vi "BMU参数读取-Auto.vi"(7 "Socket":dbl, 8 "CAN端口":u16(ring), 9 "设备索引号":u16(ring), 10 "CAN卡类型":u32(ring)=21, 11 "从板号":u8=1) -> (3 "成功?":bool)   [LabVIEW 2013] (continued)
                n1579 = Wait Until Next ms Multiple(millisecond multiple=u32 100 ("毫秒倍数")) -> ()  [unwired: 1 out]
              }
            }
            frame #2 {
              n1580 = case shown="真" w2578 {
                frame False {
                  n1581 = Concatenate Strings("故障信息" ("字符串"), "     读取失败" ("字符串")) -> (w2580:string)
                  n1582 = One Button Dialog(message=w2580, button name ("OK")="确定" ("按钮名称（“确定”）")) -> ()  [unwired: 1 out]
                }
                frame True {
                  n1583 = One Button Dialog(message="故障信息读取完成" ("字符串"), button name ("OK")="确定" ("按钮名称（“确定”）")) -> ()  [unwired: 1 out]
                }
              }
              n1584 = call <vilib>:"Unset Busy.vi"() -> ()  [unwired: 2 in, 10 out]
            }
          }
        }
        frame "平台软件版本读取" {
          n1585 = stacked-sequence {
            seq-local: [_ w2600 _] -> [_ _ w2607]
            frame #0 {
              n1586 = local read "设备索引号"() -> (w2587:u16)
              n1587 = local read "CAN卡类型"() -> (w2588:u32)
              n1588 = local read "CAN端口"() -> (w2586:u16)
              n1589 = stacked-sequence {
                tunnel: w2588 -> [w2591 w2599]
                tunnel: w2587 -> [w2590 w2598]
                tunnel: w2586 -> [w2589 w2597]
                tunnel: u8 137 ("命令") -> [_ w2596]
                frame #0 {
                  n1590 = dll-call lib="PTH1abs FBluewave New EnergySVN_WorkAutoTest_TestStandtrunkAutoTest_TestStandDriverZlgCanBHN01è¯»ååæ°data\nkerneldlls\nusbcan.dll" fn="VCI_ClearBuffer"("DeviceType"=w2591, "DeviceInd"=w2590, "CANInd"=w2589) -> (error out=w2592:errorcluster)  [unwired: 4 in, 4 out]
                  n1591 = call <vilib>:"Clear Errors.vi"("error in (no error)"=w2592) -> ()  [unwired: 6 in, 1 out]
                }
                frame #1 {
                  w2595 = u32 2 ("命令序号")
                  n1592 = local read "从板板号"() -> (w2593:u8)
                  n1593 = local write "命令"(w2596) -> ()
                  n1594 = call "多帧发送机制(EV05).vi"("can卡类型"=w2599, "设备索引号"=w2598, "CAN端口"=w2597, "命令"=w2596, "板号"=w2593, "命令序号"=w2595, "输入数据"=dbl[] [0.0]) -> ()  [unwired: 2 in, 11 out]
                  n1595 = local write "命令序号"(w2595) -> ()
                }
              }
            }
            frame #1 {
              n1596 = while {
                tunnel: [w2601] -> w2600
                i -> [w2606]
                stop <- w2603 stop-if-true
                n1597 = global read "EV05全局变量1.vi" "写入超时"() -> (w2601:bool)
                n1598 = Greater Or Equal?(x=w2606, y=25) -> (x >= y?=w2604:bool)
                n1599 = Or(x=w2601, y=w2604) -> (x .or. y?=w2603:bool)
                n1600 = Wait Until Next ms Multiple(millisecond multiple=u32 100 ("毫秒倍数")) -> ()  [unwired: 1 out]
              }
            }
            frame #2 {
              n1601 = case shown="假" w2607 {
                frame False {
                  n1602 = control-ref of="结果"() -> (w2610:refnum<vi>)
                  n1603 = Concatenate Strings("平台软件版本" ("字符串"), "     读取失败" ("字符串")) -> (w2612:string)
                  n1604 = Build Array(w2612) -> (w2609:string[])
                  n1605 = call "表格编辑(版本读取).vi"("新元素/子数组"=w2609, "活动单元格:单元格背景色"=u32 16740749, "MCListbox引用句柄"=w2610) -> ()  [unwired: 9 out]
                }
                frame True {
                }
              }
              n1606 = call <vilib>:"Unset Busy.vi"() -> ()  [unwired: 2 in, 10 out]
            }
          }
        }
        frame "模块软件版本读取" {
          n1607 = local read "从板板号"() -> (w2614:u8)
          n1608 = local read "模块软件版本"() -> (w2615:T1)
          n1609 = case shown="\"全部读取\"" w2615 {
            selector: w2615 -> [w2616 w2660]
            tunnel: w2614 -> [_ w2659]
            frame "BCUMCAL", Default {
              n1610 = stacked-sequence {
                seq-local: [_ _ w2642 _] -> [_ _ _ w2649]
                tunnel: w2616 -> [_ w2622 _ w2650]
                frame #0 {
                  w2621 = FALSE ("写?")
                  n1611 = call <vilib>:"Set Busy.vi"("disable click? (T)"=FALSE) -> ()  [unwired: 3 in, 8 out]
                  n1612 = local write "写?"(w2621) -> ()
                  n1613 = global write "EV05全局变量1.vi" "流控帧 2"(TRUE ("流控帧 2")) -> ()
                  n1614 = global write "EV05全局变量1.vi" "写入超时"(w2621) -> ()
                  n1615 = local write "控制1"(TRUE ("控制1")) -> ()
                  n1616 = local write "消除"(TRUE ("消除")) -> ()
                }
                frame #1 {
                  n1617 = Quotient & Remainder(x=w2622, y=256) -> (x-y*floor(x/y)=w2623:i32, floor(x/y)=w2624:i32)
                  n1618 = Build Array(w2624, w2623, u8 0 ("板号")) -> (w2627:i32[])
                  n1619 = local read "设备索引号"() -> (w2629:u16)
                  n1620 = local read "CAN卡类型"() -> (w2630:u32)
                  n1621 = local read "CAN端口"() -> (w2628:u16)
                  n1622 = stacked-sequence {
                    tunnel: w2630 -> [w2633 w2641]
                    tunnel: w2629 -> [w2632 w2640]
                    tunnel: w2628 -> [w2631 w2639]
                    tunnel: w2627 -> [_ w2638]
                    frame #0 {
                      n1623 = dll-call lib="PTH1abs FBluewave New EnergySVN_WorkAutoTest_TestStandtrunkAutoTest_TestStandDriverZlgCanBHN01è¯»ååæ°data\nkerneldlls\nusbcan.dll" fn="VCI_ClearBuffer"("DeviceType"=w2633, "DeviceInd"=w2632, "CANInd"=w2631) -> (error out=w2634:errorcluster)  [unwired: 4 in, 4 out]
                      n1624 = call <vilib>:"Clear Errors.vi"("error in (no error)"=w2634) -> ()  [unwired: 6 in, 1 out]
                    }
                    frame #1 {
                      w2637 = u8 137 ("命令")
                      w2635 = u32 3 ("命令序号")
                      n1625 = local read "从板板号"() -> (w2636:u8)
                      n1626 = local write "命令"(w2637) -> ()
                      n1627 = call "多帧发送机制(EV05).vi"("can卡类型"=w2641, "设备索引号"=w2640, "CAN端口"=w2639, "命令"=w2637, "板号"=w2636, "命令序号"=w2635, "输入数据"=w2638) -> ()  [unwired: 2 in, 11 out]
                      n1628 = local write "命令序号"(w2635) -> ()
                    }
                  }
                }
                frame #2 {
                  n1629 = while {
                    tunnel: [w2643] -> w2642
                    i -> [w2648]
                    stop <- w2644 stop-if-true
                    n1630 = global read "EV05全局变量1.vi" "写入超时"() -> (w2643:bool)
                    n1631 = Greater Or Equal?(x=w2648, y=25) -> (x >= y?=w2645:bool)
                    n1632 = Or(x=w2643, y=w2645) -> (x .or. y?=w2644:bool)
                    n1633 = Wait Until Next ms Multiple(millisecond multiple=u32 100 ("毫秒倍数")) -> ()  [unwired: 1 out]
                  }
                }
                frame #3 {
                  n1634 = call <vilib>:"Unset Busy.vi"() -> ()  [unwired: 2 in, 10 out]
                  n1635 = case shown="假" w2649 {
                    tunnel: w2650 -> [w2652 _]
                    frame False {
                      n1636 = Number To Decimal String(number=w2652) -> (decimal integer string=w2653:string)  [unwired: 1 out]
                      n1637 = control-ref of="结果"() -> (w2654:refnum<vi>)
                      n1638 = Concatenate Strings("模块" ("字符串"), w2653, "     读取失败" ("字符串")) -> (w2657:string)
                      n1639 = Build Array(w2657) -> (w2656:string[])
                      n1640 = call "表格编辑(版本读取).vi"("新元素/子数组"=w2656, "活动单元格:单元格背景色"=u32 16740749, "MCListbox引用句柄"=w2654) -> ()  [unwired: 9 out]
                    }
                    frame True {
                    }
                  }
                }
              }
            }
            frame "全部读取" {
              n1641 = stacked-sequence {
                seq-local: [w2661 _] -> [_ w2699]
                tunnel: w2660 -> [_ w2701]
                tunnel: w2659 -> [w2662 w2700]
                frame #0 {
                  n1642 = stacked-sequence {
                    tunnel: w2662 -> [_ w2671 _]
                    tunnel: [_ _ w2691] -> w2661
                    frame #0 {
                      w2667 = FALSE ("写?")
                      n1643 = control-ref of="模块软件版本 2"() -> (w2665:refnum<vi>)
                      n1644 = call <vilib>:"Set Busy.vi"("disable click? (T)"=FALSE) -> ()  [unwired: 3 in, 8 out]
                      n1645 = local write "写?"(w2667) -> ()
                      n1646 = property class="MCListbox (严格)"(reference=w2665, "ItemNames"=string[][] []) -> ()  [unwired: 1 in, 2 out]
                      n1647 = global write "EV05全局变量1.vi" "写入超时"(w2667) -> ()
                      n1648 = local write "消除"(TRUE ("消除")) -> ()
                      n1649 = global write "EV05全局变量1.vi" "流控帧 2"(TRUE ("流控帧 2")) -> ()
                      n1650 = local write "控制1"(TRUE ("控制1")) -> ()
                      n1651 = local write "MODEL号"(u8[] [] ("MODEL号")) -> ()
                    }
                    frame #1 {
                      n1652 = local read "设备索引号"() -> (w2673:u16)
                      n1653 = local read "CAN卡类型"() -> (w2674:u32)
                      n1654 = local read "CAN端口"() -> (w2672:u16)
                      n1655 = stacked-sequence {
                        tunnel: w2674 -> [w2677 w2690]
                        tunnel: w2673 -> [w2676 w2689]
                        tunnel: w2672 -> [w2675 w2688]
                        tunnel: w2671 -> [_ w2680]
                        frame #0 {
                          n1656 = dll-call lib="PTH1abs FBluewave New EnergySVN_WorkAutoTest_TestStandtrunkAutoTest_TestStandDriverZlgCanBHN01è¯»ååæ°data\nkerneldlls\nusbcan.dll" fn="VCI_ClearBuffer"("DeviceType"=w2677, "DeviceInd"=w2676, "CANInd"=w2675) -> (error out=w2678:errorcluster)  [unwired: 4 in, 4 out]
                          n1657 = call <vilib>:"Clear Errors.vi"("error in (no error)"=w2678) -> ()  [unwired: 6 in, 1 out]
                        }
                        frame #1 {
                          w2686 = u8 137 ("命令")
                          w2684 = u32 3 ("命令序号")
                          n1658 = Quotient & Remainder(x=u8 0 ("板号"), y=256) -> (x-y*floor(x/y)=w2681:i32, floor(x/y)=w2682:i32)
                          n1659 = local write "命令"(w2686) -> ()
                          n1660 = Build Array(w2682, w2681, u8 0 ("板号")) -> (w2687:i32[])
                          n1661 = call "多帧发送机制(EV05).vi"("can卡类型"=w2690, "设备索引号"=w2689, "CAN端口"=w2688, "命令"=w2686, "板号"=w2680, "命令序号"=w2684, "输入数据"=w2687) -> ()  [unwired: 2 in, 11 out]
                          n1662 = local write "命令序号"(w2684) -> ()
                        }
                      }
                    }
                    frame #2 {
                      n1663 = while {
                        tunnel: [w2693] -> w2691
                        i -> [w2697]
                        stop <- w2694 stop-if-true
                        n1664 = local read "强制停止版本读取"() -> (w2692:bool)
                        n1665 = global read "EV05全局变量1.vi" "写入超时"() -> (w2693:bool)
                        n1666 = Greater Or Equal?(x=w2697, y=35) -> (x >= y?=w2695:bool)
                        n1667 = Compound Arithmetic op=OR(w2692, w2693, w2695) -> (w2694:bool)
                        n1668 = Wait Until Next ms Multiple(millisecond multiple=u32 100 ("毫秒倍数")) -> ()  [unwired: 1 out]
                      }
                    }
                  }
                }
                frame #1 {
                  n1669 = case shown="真" w2699 {
                    tunnel: w2701 -> [_ w2711]
                    tunnel: w2700 -> [_ w2710]
                    frame False {
                      n1670 = control-ref of="结果"() -> (w2703:refnum<vi>)
                      n1671 = Concatenate Strings("模块编号" ("字符串"), "读取失败" ("字符串")) -> (w2706:string)
                      n1672 = Build Array(w2706) -> (w2705:string[])
                      n1673 = call "表格编辑(版本读取).vi"("新元素/子数组"=w2705, "活动单元格:单元格背景色"=u32 16740749, "MCListbox引用句柄"=w2703) -> ()  [unwired: 9 out]
                      n1674 = call <vilib>:"Unset Busy.vi"() -> ()  [unwired: 11 in, 1 out]
                    }
                    frame True {
                      n1675 = local read "MODEL号"() -> (w2709:u8[])
                      n1676 = Array Size(array=w2709) -> (size(s)=w2708:i32)
                      n1677 = for {
                        tunnel: w2711 -> [_]
                        tunnel: w2710 -> [w2714]
                        tunnel: w2709 -> [w2713] mode=indexing
                        tunnel: w2708 -> [w2712]
                        i -> [w2716]
                        n1678 = Increment(x=w2716) -> (x+1=w2715:i32)
                        n1679 = stacked-sequence {
                          seq-local: [_ _ _ w2743 _ _] -> [_ _ _ _ w2752 _]
                          seq-local: [_ w2722 _ _ _ _] -> [_ _ _ _ w2751 _]
                          tunnel: w2715 -> [_ _ _ _ _ w2763]
                          tunnel: w2713 -> [_ w2722 _ _ _ _]
                          tunnel: w2714 -> [_ w2723 _ _ _ _]
                          tunnel: w2712 -> [_ _ _ _ _ w2761]
                          frame #0 {
                            w2718 = FALSE ("写?")
                            n1680 = call <vilib>:"Set Busy.vi"("disable click? (T)"=FALSE) -> ()  [unwired: 3 in, 8 out]
                            n1681 = local write "写?"(w2718) -> ()
                            n1682 = global write "EV05全局变量1.vi" "写入超时"(w2718) -> ()
                            n1683 = global write "EV05全局变量1.vi" "流控帧 2"(TRUE ("流控帧 2")) -> ()
                            n1684 = local write "控制1"(TRUE ("控制1")) -> ()
                            n1685 = local write "消除"(TRUE ("消除")) -> ()
                          }
                          frame #1 {
                            n1686 = local read "设备索引号"() -> (w2725:u16)
                            n1687 = local read "CAN卡类型"() -> (w2726:u32)
                            n1688 = local read "CAN端口"() -> (w2724:u16)
                            n1689 = stacked-sequence {
                              tunnel: w2726 -> [w2729 w2742]
                              tunnel: w2725 -> [w2728 w2741]
                              tunnel: w2724 -> [w2727 w2740]
                              tunnel: w2723 -> [_ w2732]
                              tunnel: w2722 -> [_ w2731]
                              frame #0 {
                                n1690 = dll-call lib="PTH1abs FBluewave New EnergySVN_WorkAutoTest_TestStandtrunkAutoTest_TestStandDriverZlgCanBHN01è¯»ååæ°data\nkerneldlls\nusbcan.dll" fn="VCI_ClearBuffer"("DeviceType"=w2729, "DeviceInd"=w2728, "CANInd"=w2727) -> (error out=w2730:errorcluster)  [unwired: 4 in, 4 out]
                                n1691 = call <vilib>:"Clear Errors.vi"("error in (no error)"=w2730) -> ()  [unwired: 6 in, 1 out]
                              }
                              frame #1 {
                                w2738 = u8 137 ("命令")
                                w2736 = u32 3 ("命令序号")
                                n1692 = Quotient & Remainder(x=w2731, y=256) -> (x-y*floor(x/y)=w2733:i32, floor(x/y)=w2734:i32)
                                n1693 = local write "命令"(w2738) -> ()
                                n1694 = Build Array(w2734, w2733, u8 0 ("板号")) -> (w2739:i32[])
                                n1695 = call "多帧发送机制(EV05).vi"("can卡类型"=w2742, "设备索引号"=w2741, "CAN端口"=w2740, "命令"=w2738, "板号"=w2732, "命令序号"=w2736, "输入数据"=w2739) -> ()  [unwired: 2 in, 11 out]
                                n1696 = local write "命令序号"(w2736) -> ()
                              }
                            }
                          }
                          frame #2 {
                          }
                          frame #3 {
                            n1697 = while {
                              tunnel: [w2745] -> w2743
                              i -> [w2749]
                              stop <- w2746 stop-if-true
                              n1698 = local read "强制停止版本读取"() -> (w2744:bool)
                              n1699 = global read "EV05全局变量1.vi" "写入超时"() -> (w2745:bool)
                              n1700 = Greater Or Equal?(x=w2749, y=25) -> (x >= y?=w2747:bool)
                              n1701 = Compound Arithmetic op=OR(w2744, w2745, w2747) -> (w2746:bool)
                              n1702 = Wait Until Next ms Multiple(millisecond multiple=u32 100 ("毫秒倍数")) -> ()  [unwired: 1 out]
                            }
                          }
                          frame #4 {
                            n1703 = call <vilib>:"Unset Busy.vi"() -> ()  [unwired: 11 in, 1 out]
                            n1704 = case shown="假" w2752 {
                              tunnel: w2751 -> [w2754 _]
                              frame False {
                                n1705 = control-ref of="结果"() -> (w2756:refnum<vi>)
                                n1706 = Number To Decimal String(number=w2754) -> (decimal integer string=w2755:string)  [unwired: 1 out]
                                n1707 = Concatenate Strings("模块" ("字符串"), w2755, "     读取失败" ("字符串")) -> (w2759:string)
                                n1708 = Build Array(w2759) -> (w2758:string[])
                                n1709 = call "表格编辑(版本读取).vi"("新元素/子数组"=w2758, "活动单元格:单元格背景色"=u32 16740749, "MCListbox引用句柄"=w2756) -> ()  [unwired: 9 out]
                              }
                              frame True {
                              }
                            }
                          }
                          frame #5 {
                            n1710 = Equal?(x=w2761, y=w2763) -> (x = y?=w2762:bool)
                            n1711 = case shown="真" w2762 {
                              frame False {
                              }
                              frame True {
                                n1712 = control-ref of="模块软件版本 2"() -> (w2774:refnum<vi>)
                                n1713 = local read "模块版本名称"() -> (w2773:string[][])
                                n1714 = local read "模块版本值"() -> (w2769:string[][])
                                n1715 = control-ref of="结果"() -> (w2781:refnum<vi>)
                                n1716 = property class="MCListbox (严格)"(reference=w2774) -> ("ItemNames"=w2777:string[][])  [unwired: 1 in, 2 out]
                                n1717 = local read "从板板号"() -> (w2764:u8)
                                n1718 = Concatenate Strings("模块版本读取完成" ("字符串")) -> (w2784:string)
                                n1719 = Build Array(w2784) -> (w2783:string[])
                                n1720 = call "表格编辑(版本读取).vi"("新元素/子数组"=w2783, "活动单元格:单元格背景色"=u32 21937, "MCListbox引用句柄"=w2781) -> ()  [unwired: 9 out]
                                n1721 = Transpose 2D Array(2D array=w2777) -> (transposed array=w2778:string[][])
                                n1722 = local write "强制停止版本读取"(FALSE ("强制停止 2")) -> ()
                                n1723 = local read "模块个数"() -> (w2767:u8[])
                                n1724 = Index Array(array=w2778, index (row) #1=0 ("索引 (行)"), index (row) #2=1 ("索引 (行)")) -> (element #1=w2768:string[], element #2=w2770:string[])  [unwired: 2 in]
                                n1725 = Replace Array Subset(array=w2773, new element=w2768, index (row)=w2764) -> (w2772:string[][])  [unwired: 1 in]
                                n1726 = Replace Array Subset(array=w2769, new element=w2770, index (row)=w2764) -> (w2771:string[][])  [unwired: 1 in]
                                n1727 = local write "模块版本名称"(w2772) -> ()
                                n1728 = local write "模块版本值"(w2771) -> ()
                                n1729 = Array Size(array=w2768) -> (size(s)=w2765:i32)
                                n1730 = Replace Array Subset(array=w2767, new element=w2765, index=w2764) -> (w2766:u8[])
                                n1731 = local write "模块个数"(w2766) -> ()
                              }
                            }
                          }
                        }
                      }
                    }
                  }
                }
              }
            }
          }
        }
        frame "硬件版本读取" {
          n1732 = stacked-sequence {
            seq-local: [_ _ w2792 _] -> [_ _ _ w2799]
            frame #0 {
              w2788 = u8 137 ("命令")
              w2787 = u32 4 ("命令序号")
              n1733 = local read "设备索引号"() -> (w2790:u16)
              n1734 = local read "CAN卡类型"() -> (w2791:u32)
              n1735 = local read "CAN端口"() -> (w2789:u16)
              n1736 = local read "从板板号"() -> (w2785:u8)
              n1737 = local write "命令"(w2788) -> ()
              n1738 = call "多帧发送机制(EV05).vi"("can卡类型"=w2791, "设备索引号"=w2790, "CAN端口"=w2789, "命令"=w2788, "板号"=w2785, "命令序号"=w2787, "输入数据"=dbl[] [0.0]) -> ()  [unwired: 2 in, 11 out]
              n1739 = local write "命令序号"(w2787) -> ()
            }
            frame #1 {
            }
            frame #2 {
              n1740 = while {
                tunnel: [w2793] -> w2792
                i -> [w2798]
                stop <- w2794 stop-if-true
                n1741 = global read "EV05全局变量1.vi" "写入超时"() -> (w2793:bool)
                n1742 = Greater Or Equal?(x=w2798, y=25) -> (x >= y?=w2795:bool)
                n1743 = Or(x=w2793, y=w2795) -> (x .or. y?=w2794:bool)
                n1744 = Wait Until Next ms Multiple(millisecond multiple=u32 100 ("毫秒倍数")) -> ()  [unwired: 1 out]
              }
            }
            frame #3 {
              n1745 = case shown="假" w2799 {
                frame False {
                  n1746 = control-ref of="结果"() -> (w2801:refnum<vi>)
                  n1747 = Concatenate Strings("硬件版本" ("字符串"), "     读取失败" ("字符串")) -> (w2804:string)
                  n1748 = Build Array(w2804) -> (w2803:string[])
                  n1749 = call "表格编辑(版本读取).vi"("新元素/子数组"=w2803, "活动单元格:单元格背景色"=u32 16740749, "MCListbox引用句柄"=w2801) -> ()  [unwired: 9 out]
                }
                frame True {
                }
              }
              n1750 = call <vilib>:"Unset Busy.vi"() -> ()  [unwired: 2 in, 10 out]
            }
          }
        }
        frame "写配置文件" {
          n1751 = disable-structure shown="启用" {
            frame Enabled {
              n1752 = local read "主从选择"() -> (w2813:enum32{"主板", "从板"})
              n1753 = case shown="\"主板\", 默认" w2813 {
                tunnel: [w2832 w3023] -> w2816
                tunnel: ["M0" w3029] -> w2814
                frame "主板", Default {
                  n1754 = stacked-sequence {
                    seq-local: [w2846 _ _ _ _ _ _] -> [_ w2876 _ _ _ _ _]
                    seq-local: [string[] ["电池额定容量", "电池实际容量", "SOC", "SOH", "车牌号", "配置文件版本", "产品编号", "系统时钟"] _ _ _ _ _ _] -> [_ w2871 _ _ _ _ _]
                    seq-local: [_ _ _ _ string[] ["风机开启温度", "风机关闭温度", "加热开启温度", "加热关闭温度", "风机开启温差", "风机关闭温差", "加热关闭温差"] _ _] -> [_ _ _ _ _ w2975 _]
                    seq-local: [_ _ _ _ w2956 _ _] -> [_ _ _ _ _ w2973 _]
                    tunnel: [w2847 _ _ _ _ _ _] -> w2834
                    tunnel: [_ w2870 _ _ _ _ _] -> w2831
                    tunnel: [_ _ w2901 _ _ _ _] -> w2830
                    tunnel: [_ _ _ w2928 _ _ _] -> w2829
                    tunnel: [_ _ _ _ _ w2976 _] -> w2828
                    tunnel: [_ _ _ _ _ _ w2993] -> w2827
                    frame #0 {
                      w2838 = string[] ["", "", "", "", "", "", "", "", "", "", "  ", "", "", "", "", "", "", "", "", "", "  "]
                      n1755 = control-ref of="项目信息"() -> (w2866:refnum<vi>)
                      n1756 = property class="Tbl (严格)"(reference=w2866) -> ("Value"=w2842:string[][])  [unwired: 1 in, 2 out]
                      n1757 = control-ref of="项目信息2"() -> (w2860:refnum<vi>)
                      n1758 = Index Array(array=w2842, index (col)=0 ("禁用的索引 (列)")) -> (element=w2843:string[])  [unwired: 1 in]
                      n1759 = property class="Clust (严格)"(reference=w2860) -> ("Value"=w2859:T10)  [unwired: 1 in, 2 out]
                      n1760 = Index Array(array=w2842, index (col)=1 ("禁用的索引 (列)")) -> (element=w2841:string[])  [unwired: 1 in]
                      n1761 = local read "从板个数"() -> (w2865:dbl)
                      n1762 = Number To Decimal String(number=w2865) -> (decimal integer string=w2864:string)  [unwired: 1 out]
                      n1763 = Insert Into Array(array=w2843, new element=w2838) -> (w2840:string[])  [unwired: 1 in]
                      n1764 = Insert Into Array(array=w2841, new element=w2838) -> (w2839:string[])  [unwired: 1 in]
                      n1765 = Unbundle(w2859) -> ("电池额定容量(A)"=w2858:dbl, "电池实际容量(A)"=w2857:dbl, "车架(牌)号"=w2855:string, "配置文件版本"=w2854:string, "SOH(%)"=w2849:dbl, "SOC(%)"=w2848:dbl, "产品编号"=w2853:string, "系统时钟"=w2852:string)  [unwired: 1 out]
                      n1766 = Build Array("从板个数" ("元素"), w2864) -> (w2861:string[])
                      n1767 = Build Array(w2840, w2839) -> (w2836:string[][])
                      n1768 = Transpose 2D Array(2D array=w2836) -> (transposed array=w2835:string[][])
                      n1769 = Build Array(w2858, w2857, w2848, w2849) -> (w2856:dbl[])
                      n1770 = Build Array(w2855, w2854, w2853, w2852) -> (w2850:string[])
                      n1771 = for {
                        tunnel: w2856 -> [w2868] mode=indexing
                        tunnel: [w2867] -> w2851 mode=indexing
                        n1772 = Format Into String(format string="%#f" ("格式字符串"), w2868) -> (resulting string=w2867:string)  [unwired: 2 in, 1 out]
                      }
                      n1773 = Insert Into Array(array=w2835, index (row)=0 ("索引 (行)"), new element=w2861) -> (w2847:string[][])  [unwired: 1 in]
                      n1774 = Insert Into Array(array=w2851, new element=w2850) -> (w2846:string[])  [unwired: 1 in]
                    }
                    frame #1 {
                      n1775 = control-ref of="一级故障"() -> (w2897:refnum<vi>)
                      n1776 = property class="Clust (严格)"(reference=w2897) -> ("Value"=w2896:T11)  [unwired: 1 in, 2 out]
                      n1777 = Unbundle(w2896) -> ("总电压过高"=w2895:dbl, "整组电压不均衡"=w2890:dbl, "SOC过高"=w2883:dbl, "单体电压过高"=w2886:dbl, "总电压过低"=w2894:dbl, "温度过高"=w2893:dbl, "温度过低"=w2892:dbl, "单组电压不均衡"=w2891:dbl, "整组温度不均衡"=w2888:dbl, "单组温度不均衡"=w2889:dbl, "单体电压过低"=w2887:dbl, "充电电流过高"=w2885:dbl, "放电电流过高"=w2884:dbl, "SOC过低"=w2882:dbl, "内阻过大"=w2881:dbl, "极柱温度过高"=w2880:dbl, "SOH过低"=w2879:dbl)
                      n1778 = Build Array(w2895, w2894, w2893, w2892, w2891, w2890, w2889, w2888, w2886, w2887, w2885, w2884, w2883, w2882, w2881, w2880, w2879) -> (w2878:dbl[])
                      n1779 = for {
                        tunnel: w2878 -> [w2899] mode=indexing
                        tunnel: [w2898] -> w2875 mode=indexing
                        n1780 = Format Into String(format string="%#f" ("格式字符串"), w2899) -> (resulting string=w2898:string)  [unwired: 2 in, 1 out]
                      }
                      n1781 = Insert Into Array(array=w2876, new element=w2875) -> (w2874:string[])  [unwired: 1 in]
                      n1782 = Insert Into Array(array=w2871, new element=string[] ["总电压过高一级", "总电压过低一级", "温度过高一级", "温度过低一级", "单组电压不均衡一级", "整组电压不均衡一级", "单组温度不均衡一级", "整组温度不均衡一级", "单体电压过高一级", "单体电压过低一级", "充电电流过高一级", "放电电流过高一级", "SOC过高一级", "SOC过低一级", "内阻过大一级", "极柱温度过高一级", "SOH过低一级"]) -> (w2873:string[])  [unwired: 1 in]
                      n1783 = Build Array(w2873, w2874) -> (w2872:string[][])
                      n1784 = Transpose 2D Array(2D array=w2872) -> (transposed array=w2870:string[][])
                    }
                    frame #2 {
                      n1785 = control-ref of="一级故障 2"() -> (w2902:refnum<vi>)
                      n1786 = property class="Clust (严格)"(reference=w2902) -> ("Value"=w2924:T11)  [unwired: 1 in, 2 out]
                      n1787 = Unbundle(w2924) -> ("总电压过高"=w2923:dbl, "整组电压不均衡"=w2918:dbl, "SOC过高"=w2911:dbl, "单体电压过高"=w2914:dbl, "总电压过低"=w2922:dbl, "温度过高"=w2921:dbl, "温度过低"=w2920:dbl, "单组电压不均衡"=w2919:dbl, "整组温度不均衡"=w2916:dbl, "单组温度不均衡"=w2917:dbl, "单体电压过低"=w2915:dbl, "充电电流过高"=w2913:dbl, "放电电流过高"=w2912:dbl, "SOC过低"=w2910:dbl, "内阻过大"=w2909:dbl, "极柱温度过高"=w2908:dbl, "SOH过低"=w2907:dbl)
                      n1788 = Build Array(w2923, w2922, w2921, w2920, w2919, w2918, w2917, w2916, w2914, w2915, w2913, w2912, w2911, w2910, w2909, w2908, w2907) -> (w2906:dbl[])
                      n1789 = for {
                        tunnel: w2906 -> [w2926] mode=indexing
                        tunnel: [w2925] -> w2905 mode=indexing
                        n1790 = Format Into String(format string="%#f" ("格式字符串"), w2926) -> (resulting string=w2925:string)  [unwired: 2 in, 1 out]
                      }
                      n1791 = Build Array(string[] ["总电压过高二级", "总电压过低二级", "温度过高二级", "温度过低二级", "单组电压不均衡二级", "整组电压不均衡二级", "单组温度不均衡二级", "整组温度不均衡二级", "单体电压过高二级", "单体电压过低二级", "充电电流过高二级", "放电电流过高二级", "SOC过高二级", "SOC过低二级", "内阻过大二级", "极柱温度过高二级", "SOH过低二级"], w2905) -> (w2903:string[][])
                      n1792 = Transpose 2D Array(2D array=w2903) -> (transposed array=w2901:string[][])
                    }
                    frame #3 {
                      n1793 = control-ref of="一级故障 3"() -> (w2929:refnum<vi>)
                      n1794 = property class="Clust (严格)"(reference=w2929) -> ("Value"=w2951:T11)  [unwired: 1 in, 2 out]
                      n1795 = Unbundle(w2951) -> ("总电压过高"=w2950:dbl, "整组电压不均衡"=w2945:dbl, "SOC过高"=w2938:dbl, "单体电压过高"=w2941:dbl, "总电压过低"=w2949:dbl, "温度过高"=w2948:dbl, "温度过低"=w2947:dbl, "单组电压不均衡"=w2946:dbl, "整组温度不均衡"=w2943:dbl, "单组温度不均衡"=w2944:dbl, "单体电压过低"=w2942:dbl, "充电电流过高"=w2940:dbl, "放电电流过高"=w2939:dbl, "SOC过低"=w2937:dbl, "内阻过大"=w2936:dbl, "极柱温度过高"=w2935:dbl, "SOH过低"=w2934:dbl)
                      n1796 = Build Array(w2950, w2949, w2948, w2947, w2946, w2945, w2944, w2943, w2941, w2942, w2940, w2939, w2938, w2937, w2936, w2935, w2934) -> (w2933:dbl[])
                      n1797 = for {
                        tunnel: w2933 -> [w2953] mode=indexing
                        tunnel: [w2952] -> w2932 mode=indexing
                        n1798 = Format Into String(format string="%#f" ("格式字符串"), w2953) -> (resulting string=w2952:string)  [unwired: 2 in, 1 out]
                      }
                      n1799 = Build Array(string[] ["总电压过高三级", "总电压过低三级", "温度过高三级", "温度过低三级", "单组电压不均衡三级", "整组电压不均衡三级", "单组温度不均衡三级", "整组温度不均衡三级", "单体电压过高三级", "单体电压过低三级", "充电电流过高三级", "放电电流过高三级", "SOC过高三级", "SOC过低三级", "内阻过大三级", "极柱温度过高三级", "SOH过低三级"], w2932) -> (w2930:string[][])
                      n1800 = Transpose 2D Array(2D array=w2930) -> (transposed array=w2928:string[][])
                    }
                    frame #4 {
                      n1801 = control-ref of="加热控制参数"() -> (w2966:refnum<vi>)
                      n1802 = property class="Clust (严格)"(reference=w2966) -> ("Value"=w2965:T12)  [unwired: 1 in, 2 out]
                      n1803 = Unbundle(w2965) -> ("风机开启温度"=w2964:dbl, "风机关闭温度"=w2963:dbl, "加热开启温度"=w2962:dbl, "加热关闭温度"=w2961:dbl, "风机开启温差"=w2960:dbl, "风机关闭温差"=w2959:dbl, "加热关闭温差"=w2955:dbl)
                      n1804 = Build Array(w2964, w2963, w2962, w2961, w2960, w2959, w2955) -> (w2958:dbl[])
                      n1805 = for {
                        tunnel: w2958 -> [w2968] mode=indexing
                        tunnel: [w2967] -> w2956 mode=indexing
                        n1806 = Format Into String(format string="%#f" ("格式字符串"), w2968) -> (resulting string=w2967:string)  [unwired: 2 in, 1 out]
                      }
                    }
                    frame #5 {
                      n1807 = control-ref of="充电控制参数"() -> (w2986:refnum<vi>)
                      n1808 = property class="Clust (严格)"(reference=w2986) -> ("Value"=w2988:T13)  [unwired: 1 in, 2 out]
                      n1809 = Unbundle(w2988) -> ("最大允许单体电压"=w2985:dbl, "最大允许总电压"=w2984:dbl, "最小允许单体电压"=w2983:dbl, "最大允许充电电流"=w2982:dbl, "最小允许充电电流"=w2981:dbl, "最大允许充电温度"=w2980:dbl, "最小允许充电温度"=w2979:dbl, "电流步长"=w2978:dbl)
                      n1810 = Build Array(w2985, w2984, w2983, w2982, w2981, w2980, w2979, w2978) -> (w2987:dbl[])
                      n1811 = for {
                        tunnel: w2987 -> [w2990] mode=indexing
                        tunnel: [w2989] -> w2972 mode=indexing
                        n1812 = Format Into String(format string="%#f" ("格式字符串"), w2990) -> (resulting string=w2989:string)  [unwired: 2 in, 1 out]
                      }
                      n1813 = Insert Into Array(array=w2973, new element=w2972) -> (w2971:string[])  [unwired: 1 in]
                      n1814 = Insert Into Array(array=w2975, new element=string[] ["最大允许单体电压", "最大允许总电压", "最小允许单体电压", "最大允许充电电流", "最小允许充电电流", "最大允许充电温度", "最小允许充电温度", "电流步长"]) -> (w2970:string[])  [unwired: 1 in]
                      n1815 = Build Array(w2970, w2971) -> (w2977:string[][])
                      n1816 = Transpose 2D Array(2D array=w2977) -> (transposed array=w2976:string[][])
                    }
                    frame #6 {
                      n1817 = control-ref of="电池信息"() -> (w3014:refnum<vi>)
                      n1818 = property class="Clust (严格)"(reference=w3014) -> ("Value"=w3017:T14)  [unwired: 1 in, 2 out]
                      n1819 = Unbundle(w3017) -> ("电池串联"=w3013:dbl, "电池并联"=w3012:dbl, "累计放电总安时"=w3010:dbl, "电池包额定容量"=w3009:dbl, "电池包额定能量(kWh)"=w3008:dbl, "电池包额定总电压"=w3007:dbl, "累计充电总安时"=w3011:dbl, "电池充满次数"=w3006:dbl, "电池放空次数"=w3005:dbl, "电池充电次数"=w3004:dbl, "电池生产日期"=w3002:string, "电池厂家"=w3001:string, "电池类型"=w3000:string, "电池包组号"=w2999:string, "电池包产权标识"=w2998:string, "电池应用车型"=w2997:string, "实际容量"=w2992:dbl)
                      n1820 = Build Array(w3002, w3001, w3000, w2999, w2998, w2997) -> (w2996:string[])
                      n1821 = Build Array(w3013, w3012, w3011, w3010, w3009, w3008, w3007, w3006, w3005, w3004, w2992) -> (w3003:dbl[])
                      n1822 = for {
                        tunnel: w3003 -> [w3019] mode=indexing
                        tunnel: [w3018] -> w2995 mode=indexing
                        n1823 = Format Into String(format string="%#f" ("格式字符串"), w3019) -> (resulting string=w3018:string)  [unwired: 2 in, 1 out]
                      }
                      n1824 = Insert Into Array(array=w2996, new element=w2995) -> (w2994:string[])  [unwired: 1 in]
                      n1825 = call <vilib>:"Unset Busy.vi"() -> ()  [unwired: 2 in, 10 out]
                      n1826 = Build Array(string[] ["电池生产日期", "电池厂商", "电池类型", "电池包组号", "电池包产权标识", "电池包应用车型", "电池串联", "电池并联", "累计充电总安时", "累计放电总安时", "电池包额定容量", "电池包额定能量", "电池包额定总电压", "电池充满次数", "电池放空次数", "电池充电次数", "实际容量"], w2994) -> (w3015:string[][])
                      n1827 = Transpose 2D Array(2D array=w3015) -> (transposed array=w2993:string[][])
                    }
                  }
                  n1828 = Insert Into Array(array=w2834, index (col)=2 ("禁用的索引 (列)"), new element #1=w2831, new element #2=w2830, new element #3=w2829, new element #4=w2828, new element #5=w2827) -> (w2832:string[][])  [unwired: 1 in]
                }
                frame "从板" {
                  n1829 = local read "从板号"() -> (w3031:u8)
                  n1830 = Number To Decimal String(number=w3031) -> (decimal integer string=w3028:string)  [unwired: 1 out]
                  n1831 = Concatenate Strings("S", w3028) -> (w3029:string)
                  n1832 = Build Array("从板号" ("元素"), w3028) -> (w3026:string[])
                  n1833 = stacked-sequence {
                    seq-local: [string[] ["风机开启温度", "风机关闭温度", "加热开启温度", "加热关闭温度", "风机开启温差", "风机关闭温差", "加热关闭温差"] _ _ _ _ _] -> [_ _ _ w3100 _ _]
                    seq-local: [w3043 _ _ _ _ _] -> [_ _ _ w3096 _ _]
                    seq-local: [_ string[] ["电压过高一级", "电压过低一级", "温度过高一级", "温度过低一级", "电压不均衡一级", "温度不均衡一级", "SOC过低一级"] _ _ _ _] -> [_ _ _ w3099 _ _]
                    seq-local: [_ w3061 _ _ _ _] -> [_ _ _ w3095 _ _]
                    seq-local: [_ _ string[] ["电压过高二级", "电压过低二级", "温度过高二级", "温度过低二级", "电压不均衡二级", "温度不均衡二级", "SOC过低二级"] _ _ _] -> [_ _ _ w3098 _ _]
                    seq-local: [_ _ w3076 _ _ _] -> [_ _ _ w3094 _ _]
                    tunnel: w3026 -> [w3056 _ _ _ _ _]
                    tunnel: [w3045 _ _ _ _ _] -> w3024
                    tunnel: [_ _ _ w3101 _ _] -> w3022
                    tunnel: [_ _ _ _ w3139 _] -> w3021
                    tunnel: [_ _ _ _ _ w3175] -> _
                    frame #0 {
                      w3036 = string[] ["", "", "", "", "", "", "", "", "", "", "  "]
                      n1834 = control-ref of="项目信息 2"() -> (w3055:refnum<vi>)
                      n1835 = property class="Tbl (严格)"(reference=w3055) -> ("Value"=w3033:string[][])  [unwired: 1 in, 2 out]
                      n1836 = control-ref of="加热控制参数"() -> (w3047:refnum<vi>)
                      n1837 = property class="Clust (严格)"(reference=w3047) -> ("Value"=w3054:T12)  [unwired: 1 in, 2 out]
                      n1838 = Unbundle(w3054) -> ("风机开启温度"=w3053:dbl, "风机关闭温度"=w3052:dbl, "加热开启温度"=w3051:dbl, "加热关闭温度"=w3050:dbl, "风机开启温差"=w3049:dbl, "风机关闭温差"=w3048:dbl, "加热关闭温差"=w3042:dbl)
                      n1839 = Build Array(w3053, w3052, w3051, w3050, w3049, w3048, w3042) -> (w3046:dbl[])
                      n1840 = for {
                        tunnel: w3046 -> [w3059] mode=indexing
                        tunnel: [w3058] -> w3043 mode=indexing
                        n1841 = Format Into String(format string="%#f" ("格式字符串"), w3059) -> (resulting string=w3058:string)  [unwired: 2 in, 1 out]
                      }
                      n1842 = Index Array(array=w3033, index (col)=0 ("禁用的索引 (列)")) -> (element=w3040:string[])  [unwired: 1 in]
                      n1843 = Index Array(array=w3033, index (col)=1 ("禁用的索引 (列)")) -> (element=w3039:string[])  [unwired: 1 in]
                      n1844 = Insert Into Array(array=w3040, new element=w3036) -> (w3038:string[])  [unwired: 1 in]
                      n1845 = Insert Into Array(array=w3039, new element=w3036) -> (w3037:string[])  [unwired: 1 in]
                      n1846 = Build Array(w3038, w3037) -> (w3034:string[][])
                      n1847 = Transpose 2D Array(2D array=w3034) -> (transposed array=w3032:string[][])
                      n1848 = Insert Into Array(array=w3032, index (row)=0 ("索引 (行)"), new element=w3056) -> (w3045:string[][])  [unwired: 1 in]
                    }
                    frame #1 {
                      n1849 = control-ref of="一级故障(从板)"() -> (w3072:refnum<vi>)
                      n1850 = property class="Clust (严格)"(reference=w3072) -> ("Value"=w3071:T16)  [unwired: 1 in, 2 out]
                      n1851 = Unbundle(w3071) -> ("电压过高"=w3070:dbl, "电压过低"=w3069:dbl, "温度过高"=w3068:dbl, "温度过低"=w3067:dbl, "电压不均衡(V)"=w3066:dbl, "温度不均衡"=w3065:dbl, "SOC过低"=w3064:dbl)
                      n1852 = Build Array(w3070, w3069, w3068, w3067, w3066, w3065, w3064) -> (w3063:dbl[])
                      n1853 = for {
                        tunnel: w3063 -> [w3074] mode=indexing
                        tunnel: [w3073] -> w3061 mode=indexing
                        n1854 = Format Into String(format string="%#f" ("格式字符串"), w3074) -> (resulting string=w3073:string)  [unwired: 2 in, 1 out]
                      }
                    }
                    frame #2 {
                      n1855 = control-ref of="二级故障(从板)"() -> (w3078:refnum<vi>)
                      n1856 = property class="Clust (严格)"(reference=w3078) -> ("Value"=w3087:T16)  [unwired: 1 in, 2 out]
                      n1857 = Unbundle(w3087) -> ("电压过高"=w3086:dbl, "电压过低"=w3085:dbl, "温度过高"=w3084:dbl, "温度过低"=w3083:dbl, "电压不均衡(V)"=w3082:dbl, "温度不均衡"=w3081:dbl, "SOC过低"=w3080:dbl)
                      n1858 = Build Array(w3086, w3085, w3084, w3083, w3082, w3081, w3080) -> (w3079:dbl[])
                      n1859 = for {
                        tunnel: w3079 -> [w3089] mode=indexing
                        tunnel: [w3088] -> w3076 mode=indexing
                        n1860 = Format Into String(format string="%#f" ("格式字符串"), w3089) -> (resulting string=w3088:string)  [unwired: 2 in, 1 out]
                      }
                    }
                    frame #3 {
                      n1861 = control-ref of="三级故障(从板)"() -> (w3102:refnum<vi>)
                      n1862 = property class="Clust (严格)"(reference=w3102) -> ("Value"=w3112:T16)  [unwired: 1 in, 2 out]
                      n1863 = Unbundle(w3112) -> ("电压过高"=w3111:dbl, "电压过低"=w3110:dbl, "温度过高"=w3109:dbl, "温度过低"=w3108:dbl, "电压不均衡(V)"=w3107:dbl, "温度不均衡"=w3106:dbl, "SOC过低"=w3105:dbl)
                      n1864 = Build Array(w3111, w3110, w3109, w3108, w3107, w3106, w3105) -> (w3104:dbl[])
                      n1865 = for {
                        tunnel: w3104 -> [w3114] mode=indexing
                        tunnel: [w3113] -> w3093 mode=indexing
                        n1866 = Format Into String(format string="%#f" ("格式字符串"), w3114) -> (resulting string=w3113:string)  [unwired: 2 in, 1 out]
                      }
                      n1867 = Insert Into Array(array=w3100, new element #1=w3099, new element #2=w3098, new element #3=string[] ["电压过高三级", "电压过低三级", "温度过高三级", "温度过低三级", "电压不均衡三级", "温度不均衡三级", "SOC过低三级"]) -> (w3091:string[])  [unwired: 1 in]
                      n1868 = Insert Into Array(array=w3096, new element #1=w3095, new element #2=w3094, new element #3=w3093) -> (w3092:string[])  [unwired: 1 in]
                      n1869 = Build Array(w3091, w3092) -> (w3103:string[][])
                      n1870 = Transpose 2D Array(2D array=w3103) -> (transposed array=w3101:string[][])
                    }
                    frame #4 {
                      n1871 = control-ref of="快换(从板)"() -> (w3138:refnum<vi>)
                      n1872 = property class="Clust (严格)"(reference=w3138) -> ("Value"=w3151:T17)  [unwired: 1 in, 2 out]
                      n1873 = Unbundle(w3151) -> ("串联数"=w3150:dbl, "并联数"=w3149:dbl, "电池厂家"=w3148:dbl, "电池类型"=w3147:dbl, "额定能量"=w3146:dbl, "额定容量"=w3145:dbl, "实际容量"=w3144:dbl, "额定总压"=w3137:dbl, "产权标识"=w3136:dbl, "应用车型"=w3135:dbl, "电池包组号"=w3134:dbl, "SOC"=w3132:dbl, "充电总安时"=w3131:dbl, "放电总安时"=w3130:dbl, "放空次数"=w3129:dbl, "充满次数"=w3128:dbl, "充电次数"=w3127:dbl, "车牌号"=w3117:string, "生产日期"=w3116:string, "最大允许单体电压"=w3126:dbl, "最大允许总电压"=w3125:dbl, "最大允许温度"=w3124:dbl, "最小允许温度"=w3123:dbl, "最大允许充电电流"=w3122:dbl, "最小允许充电电流"=w3121:dbl, "最小允许单体电压"=w3120:dbl, "电流步长"=w3119:dbl, "电池包序号"=w3118:dbl)
                      n1874 = Build Array(w3150, w3149, w3148, w3147, w3146, w3145, w3144, w3137, w3136, w3135, w3134, w3132, w3131, w3130, w3129, w3128, w3127, w3126, w3125, w3124, w3123, w3122, w3121, w3120, w3119, w3118) -> (w3143:dbl[])
                      n1875 = for {
                        tunnel: w3143 -> [w3153] mode=indexing
                        tunnel: [w3152] -> w3141 mode=indexing
                        n1876 = Format Into String(format string="%#f" ("格式字符串"), w3153) -> (resulting string=w3152:string)  [unwired: 2 in, 1 out]
                      }
                      n1877 = Insert Into Array(array=w3141, new element #1=w3117, new element #2=w3116) -> (w3133:string[])  [unwired: 1 in]
                      n1878 = call <vilib>:"Unset Busy.vi"() -> ()  [unwired: 2 in, 10 out]
                      n1879 = Build Array(string[] ["电池串联数", "电池并联数", "电池厂家", "额定能量", "额定容量", "实际容量", "额定总压", "产权标识", "应用车型", "电池包组号", "SOC", "充电总安时", "放电总安时", "放空次数", "充满次数", "充电次数", "最大允许单体电压", "最大允许总电压", "最大允许温度", "最小允许温度", "最大允许充电电流", "最小允许充电电流", "最小允许单体电压", "电流步长", "电池包序号"], w3133) -> (w3142:string[][])
                      n1880 = Transpose 2D Array(2D array=w3142) -> (transposed array=w3139:string[][])
                    }
                    frame #5 {
                      n1881 = local read "均衡参数"() -> (w3174:T18)
                      n1882 = Unbundle(w3174) -> ("充电结束电压(90%)"=w3166:sgl, "充电结束电压(91%)"=w3165:sgl, "充电结束电压(92%)"=w3164:sgl, "充电结束电压(93%)"=w3163:sgl, "充电结束电压(94%)"=w3162:sgl, "均衡计算-电压高阀值1级"=w3173:sgl, "均衡计算-电压高阀值2级"=w3172:sgl, "均衡计算-电压低阀值1级"=w3171:sgl, "均衡计算-电压低阀值2级"=w3170:sgl, "均衡计算-最低电压阀值"=w3169:sgl, "均衡停止-最低电压阀值"=w3168:sgl, "均衡计算-电压极差阀值"=w3167:sgl, "充电结束电压(95%)"=w3161:sgl, "充电结束电压(96%)"=w3160:sgl, "充电结束电压(97%)"=w3159:sgl, "充电结束电压(98%)"=w3158:sgl, "充电结束电压(99%)"=w3157:sgl, "充电结束电压(100%)"=w3156:sgl)
                      n1883 = Build Array(w3173, w3172, w3171, w3170, w3169, w3168, w3167, w3166, w3165, w3164, w3163, w3162, w3161, w3160, w3159, w3158, w3157, w3156) -> (w3178:sgl[])
                      n1884 = for {
                        tunnel: w3178 -> [w3180] mode=indexing
                        tunnel: [w3179] -> w3155 mode=indexing
                        n1885 = Format Into String(format string="%#f" ("格式字符串"), w3180) -> (resulting string=w3179:string)  [unwired: 2 in, 1 out]
                      }
                      n1886 = call <vilib>:"Unset Busy.vi"() -> ()  [unwired: 2 in, 10 out]
                      n1887 = Build Array(string[] ["均衡计算-电压高阀值1级", "均衡计算-电压高阀值2级", "均衡计算-电压低阀值1级", "均衡计算-电压低阀值2级", "均衡计算-最低电压阀值", "均衡停止-最低电压阀值", "均衡计算-电压极差阀值", "充电结束电压(90%)", "充电结束电压(91%)", "充电结束电压(92%)", "充电结束电压(93%)", "充电结束电压(94%)", "充电结束电压(95%)", "充电结束电压(96%)", "充电结束电压(97%)", "充电结束电压(98%)", "充电结束电压(99%)", "充电结束电压(100%)"], w3155) -> (w3177:string[][])
                      n1888 = Transpose 2D Array(2D array=w3177) -> (transposed array=w3175:string[][])
                    }
                  }
                  n1889 = Insert Into Array(array=w3024, index (col)=2 ("禁用的索引 (列)"), new element #1=w3022, new element #2=w3021) -> (w3023:string[][])  [unwired: 1 in]
                }
              }
              n1890 = call "当前时间解析-8.6.vi"() -> ("名称格式时间"=w2815:string)  [unwired: 1 in, 18 out]
              n1891 = Concatenate Strings(w2815, w2814, ".txt" ("字符串")) -> (w2812:string)
              n1892 = call "自适应屏幕分辨率.vi"() -> ()  [unwired: 16 in]
              n1893 = call "文件对话框2"("prompt"="选择保存的路径", "default name"=w2812, "pattern (all files)"="*.txt") -> ("selected path"=w2810:path, "cancelled"=w2809:bool, "error out"=w2808:errorcluster)  [unwired: 9 in, 1 out]
              n1894 = call <vilib>:"Clear Errors.vi"("error in (no error)"=w2808) -> ()  [unwired: 6 in, 1 out]
              n1895 = case shown="假" w2809 {
                tunnel: w2816 -> [w2821 _]
                tunnel: w2810 -> [w2817 _]
                frame False {
                  n1896 = call-poly <vilib>:"Write To Spreadsheet File.vi"("append to file? (new file:F)"=FALSE, "2D data"=w2821, "file path (dialog if empty)"=w2817) -> ("new file path (Not A Path if cancelled)"=w2819:path)  [unwired: 3 in, 2 out]
                  n1897 = Path To String(path=w2819) -> (string=w2818:string)
                  n1898 = stacked-sequence {
                    tunnel: w2818 -> [w2824]
                    frame #0 {
                      n1899 = Concatenate Strings("保存完成,路径为:" ("字符串"), w2824) -> (w2825:string)
                      n1900 = One Button Dialog(message=w2825, button name ("OK")="是" ("按钮名称（“确定”）")) -> ()  [unwired: 1 out]
                    }
                  }
                }
                frame True {
                }
              }
            }
            frame Disabled {
              n1901 = stacked-sequence {
                seq-local: [w3195] -> [_]
                frame #0 {
                  n1902 = local read "项目信息"() -> (w3197:string[][])
                  n1903 = local read "项目信息2"() -> (w3194:T10)
                  n1904 = Array Subset(array=w3197, index (row)=0 ("索引"), index (col)=0 ("索引"), length (col)=2 ("索引")) -> (w3200:string[][])  [unwired: 1 in]
                  n1905 = local read "一级故障"() -> ()  [unwired: 1 out]
                  n1906 = local read "从板个数"() -> (w3195:dbl)
                  n1907 = Unbundle(w3194) -> ("电池额定容量(A)"=w3193:dbl, "电池实际容量(A)"=w3192:dbl, "车架(牌)号"=w3186:string, "配置文件版本"=w3185:string, "SOH(%)"=w3190:dbl, "SOC(%)"=w3191:dbl, "产品编号"=w3187:string)  [unwired: 2 out]
                  n1908 = Index Array(array=w3200, index (col) #1=1 ("禁用的索引 (列)"), index (col) #2=0 ("索引 (列)")) -> (element #1=w3184:string[], element #2=w3183:string[])  [unwired: 2 in]
                  n1909 = Build Array(w3193, w3192, w3191, w3190) -> (w3189:dbl[])
                  n1910 = Number To Decimal String(number=w3195) -> ()  [unwired: 1 in, 1 out]
                  n1911 = for {
                    tunnel: w3189 -> [w3205] mode=indexing
                    tunnel: [w3204] -> w3188 mode=indexing
                    n1912 = Format Into String(format string="%#f" ("格式字符串"), w3205) -> (resulting string=w3204:string)  [unwired: 2 in, 1 out]
                  }
                  n1913 = Insert Into Array(array=w3188, new element #1=w3187, new element #2=w3186, new element #3=w3185, new element #4=w3184) -> ()  [unwired: 1 in, 1 out]
                  n1914 = Insert Into Array(array=string[] ["电池额定容量", "电池实际容量", "SOC", "SOH", "产品编号", "车架(牌)号", "配置文件版本"], new element=w3183) -> ()  [unwired: 1 in, 1 out]
                }
              }
            }
          }
        }
        frame "读配置文件" {
        }
      }
    }
    frame Error {
    }
  }
  n1915 = while {
    tunnel: w31 -> [w3217]
    tunnel: w30 -> [w3216]
    tunnel: [w3215] -> w34
    tunnel: [w3214] -> w33
    tunnel: w26 -> [_]
    tunnel: w29 -> [w3206]
    stop <- w3213 stop-if-true
    n1916 = local read "停止"() -> (w3213:bool)
    n1917 = local read "设备索引号"() -> (w3210:u16)
    n1918 = local read "CAN卡类型"() -> (w3211:u32)
    n1919 = local read "CAN端口"() -> (w3209:u16)
    n1920 = call "receiver-8.6.vi"("错误输入（无错误）"=w3206, "CAN端口"=w3209, "设备索引号"=w3210, "CAN卡类型"=w3211) -> ("错误输出"=w3212:errorcluster, "输出簇"=w3208:T28, "接收成功"=w3207:bool)  [unwired: 3 out]
    n1921 = call <vilib>:"Clear Errors.vi"("error in (no error)"=w3212) -> ()  [unwired: 6 in, 1 out]
    n1922 = case shown="真" w3207 {
      tunnel: w3216 -> [w3218 w3224]
      tunnel: w3208 -> [_ w3223]
      tunnel: w3217 -> [w3219 w3222]
      tunnel: [w3219 w3221] -> w3215
      tunnel: [w3218 w3220] -> w3214
      frame False {
      }
      frame True {
        n1923 = Enqueue Element(queue=w3222, element=w3223, error in (no error)=w3224) -> (queue out=w3221:refnum<queue>, error out=w3220:errorcluster)  [unwired: 2 out]
      }
    }
  }
  n1924 = while {
    tunnel: w31 -> [w3232]
    tunnel: w30 -> [w3231]
    stop <- w3225 stop-if-true
    n1925 = local read "停止"() -> (w3225:bool)
    n1926 = local read "控制1"() -> (w3227:bool)
    n1927 = Dequeue Element(queue=w3232, timeout in ms (-1)=200 ("超时毫秒(-1)"), error in (no error)=w3231) -> (element=w3230:T3, error out=w3229:errorcluster)  [unwired: 2 out]
    n1928 = case shown="无错误" w3229 {
      tunnel: w3230 -> [w3237 _]
      tunnel: "写?" -> [w3234 _]
      tunnel: w3227 -> [w3233 _]
      frame No Error {
        n1929 = Unbundle(w3237) -> ("return type"=w3236:u32, "pReceive"=w3235:T29)
        n1930 = for {
          N: w3236 -> [_]
          tunnel: w3235 -> [w3241] mode=indexing
          tunnel: w3234 -> [w3239]
          tunnel: w3233 -> [w3238]
          n1931 = Unbundle By Name(w3241) -> ("ID"=w3242:u32)
          n1932 = call "ID解析.vi"("ID"=w3242) -> ("PDU(1)"=w3240:i32)  [unwired: 10 out]
          n1933 = case shown="18" w3240 {
            tunnel: w3241 -> [_ w3252]
            tunnel: w3239 -> [_ w3244]
            tunnel: w3238 -> [_ w3243]
            frame 0, Default {
            }
            frame 24 {
              n1934 = local read "主从选择"() -> (w3245:enum32{"主板", "从板"})
              n1935 = local read "设备索引号"() -> (w3248:u16)
              n1936 = local read "CAN卡类型"() -> (w3247:u32)
              n1937 = local read "CAN端口"() -> (w3249:u16)
              n1938 = disable-structure shown="禁用" {
                disable-tunnel: w3252 -> [w3255 _]
                frame Disabled {
                  n1939 = call "标定授权读取.vi"("VCI_Receive"=w3255) -> ()  [unwired: 1 out]
                }
                frame Enabled {
                }
              }
              n1940 = case shown="\"主板\", 默认" w3245 {
                tunnel: [0 ("FUNC") w3254] -> w3246
                frame "主板", Default {
                }
                frame "从板" {
                  n1941 = local read "从板号"() -> (w3254:u8)
                }
              }
              n1942 = local read "面板选择"() -> (w3251:T7)
              n1943 = case shown="\"读写参数\", 默认" w3251 {
                tunnel: w3244 -> [w3262 _ _ _]
                tunnel: "命令" -> [w3263 w3368 w3623 w3763]
                tunnel: w3245 -> [w3272 _ w3631 w3771]
                tunnel: w3252 -> [_ _ _ _]
                tunnel: w3252 -> [w3268 w3369 w3625 w3765]
                tunnel: w3249 -> [w3267 w3370 w3626 w3766]
                tunnel: w3248 -> [w3266 w3371 w3627 w3767]
                tunnel: w3247 -> [w3265 w3372 w3628 w3768]
                tunnel: w3246 -> [w3264 _ w3624 w3764]
                tunnel: w3243 -> [w3258 _ _ _]
                frame "读写参数", Default {
                  n1944 = control-ref of="流控帧 2"() -> (w3256:refnum<vi>)
                  n1945 = control-ref of="流控帧"() -> (w3257:refnum<vi>)
                  n1946 = local read "命令序号"() -> (w3261:u8)
                  n1947 = call "多帧接收机制(EV05).vi"("can卡类型"=w3265, "设备索引号"=w3266, "CAN端口"=w3267, "VCI_Receive"=w3268, "命令"=w3263, "板号"=w3264, "流控帧"=w3257, "写?"=w3262, "流控帧2"=w3256, "命令序号"=w3261) -> ("错误信号"=w3259:bool, "错误代码"=w3271:i32, "输出数组"=w3270:u8[], "读错误代码"=w3260:u8[], "结束信号"=w3269:bool)  [unwired: 5 out]
                  n1948 = case shown="假" w3262 {
                    tunnel: w3269 -> [w3282 w3351]
                    tunnel: w3271 -> [w3281 w3350]
                    tunnel: w3261 -> [w3280 _]
                    tunnel: w3270 -> [w3279 _]
                    tunnel: w3263 -> [w3278 _]
                    tunnel: w3272 -> [w3276 w3349]
                    tunnel: w3260 -> [w3275 _]
                    tunnel: w3259 -> [w3274 _]
                    tunnel: w3258 -> [w3273 _]
                    frame False {
                      # "读参数"
                      n1949 = And(x=w3273, y=w3282) -> (x .and. y?=w3277:bool)
                      n1950 = case shown="真" w3277 {
                        tunnel: w3281 -> [_ w3293]
                        tunnel: w3280 -> [_ w3292]
                        tunnel: w3279 -> [_ w3291]
                        tunnel: w3278 -> [_ w3290]
                        tunnel: w3276 -> [_ w3286]
                        tunnel: w3275 -> [_ w3284]
                        tunnel: w3274 -> [_ w3285]
                        frame False {
                        }
                        frame True {
                          n1951 = case shown="假" w3285 {
                            tunnel: w3293 -> [w3306 _]
                            tunnel: w3292 -> [w3305 _]
                            tunnel: w3291 -> [w3304 _]
                            tunnel: w3290 -> [w3302 _]
                            tunnel: w3286 -> [w3298 _]
                            tunnel: w3284 -> [_ w3334]
                            frame False {
                              n1952 = case shown="\"主板\", 默认" w3298 {
                                tunnel: [w3308 _] -> w3301
                                tunnel: [_ w3322] -> w3300
                                tunnel: [w3307 _] -> w3297
                                frame "主板", Default {
                                n1953 = stacked-sequence {
                                tunnel: [_ w3321] -> w3308
                                tunnel: [w3309 _] -> w3307
                                frame #0 {
                                n1954 = control-ref of="一级故障"() -> (w3315:refnum<vi>)
                                n1955 = control-ref of="一级故障 2"() -> (w3317:refnum<vi>)
                                n1956 = control-ref of="一级故障 3"() -> (w3318:refnum<vi>)
                                n1957 = control-ref of="加热控制参数"() -> (w3319:refnum<vi>)
                                n1958 = control-ref of="充电控制参数"() -> (w3320:refnum<vi>)
                                n1959 = control-ref of="电池信息"() -> (w3313:refnum<vi>)
                                n1960 = control-ref of="项目信息"() -> (w3316:refnum<vi>)
                                n1961 = control-ref of="项目信息2"() -> (w3314:refnum<vi>)
                                n1962 = control-ref of="高压参数"() -> (w3312:refnum<vi>)
                                n1963 = local read "主板数据"() -> (w3311:T4)
                                n1964 = Bundle(cluster=w3311, "项目信息"=w3316, "一级故障 4"=w3314, "一级故障"=w3315, "一级故障 2"=w3317, "一级故障 3"=w3318, "加热控制参数"=w3319, "充电控制参数"=w3320, "高压参数"=w3312, "电池信息"=w3313) -> (w3310:T4)
